vi "TRIM-BOTH-SPACE.vi"(3 "name in":string) -> (1 "name out":string)   [LabVIEW 2014, in "TagDB(dev).lvlib"]
uses:
  TagDB(dev).lvlib
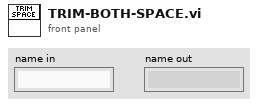
[diagram p1: front panel]
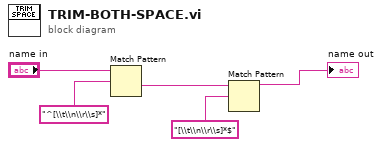
[diagram p0: block diagram]
diagram:
  n1 = Match Pattern(string="name in", regular expression="^[\\t\\n\\r\\s]*") -> (after substring=w4:string)  [unwired: 1 in, 3 out]
  n2 = Match Pattern(string=w4, regular expression="[\\t\\n\\r\\s]*$") -> (before substring=→"name out":string)  [unwired: 1 in, 3 out]
